vi "Periodic Tasks.vi"(8 "error in":errorcluster) -> ()   [LabVIEW 2017]
doc: "This VI runs in parallel to other tasks. It can contain as many user-defined periodic loops as you need. These can carry out PID or other sorts of timed response."
uses:
  Public/Documents/Cross The Road Electronics/Phoenix-LabVIEW/Motor Controller/Controls/CTRE_Phoenix_MotorControl_ControlMode.ctl
  Public/Documents/Cross The Road Electronics/Phoenix-LabVIEW/Motor Controller/Controls/CTRE_Phoenix_MotorControl_FeedbackDevice.ctl
  <vilib>/Rock Robotics/WPI/Utilities/WPI_GetSetVariantRefNum.vi
  Public/Documents/Cross The Road Electronics/Phoenix-LabVIEW/Motor Controller/Get/CTRE_Phoenix_MotorController_GetSelectedSensorData.vi
  Public/Documents/Cross The Road Electronics/Phoenix-LabVIEW/Motor Controller/Get/CTRE_Phoenix_MotorController_GetClosedLoopData.vi
panel:
  out "Error":T1(graph)
  in  "Left Phase":bool
  in  "Right Phase":bool
  in  "Setpoint":dbl
  in  "Control Mode":T2 items=["PercentOutput"=0, "Position"=1, "Velocity"=2, "Current"=3, "Follower"=5, "MotionProfile"=6, "MotionMagic"=7, "MotionMagicArc"=8, "MotionProfileArc"=10, "Disabled"=15]
  in  "Run PID":bool
  in  "Motion Magic":T3
  in  "Constants":cluster{"P":dbl, "I":dbl, "D":dbl, "F":dbl}
  in  "Change PID Constants":bool=TRUE
  in  "Zero Drive Sensors":bool
  out "Position":T4(graph)
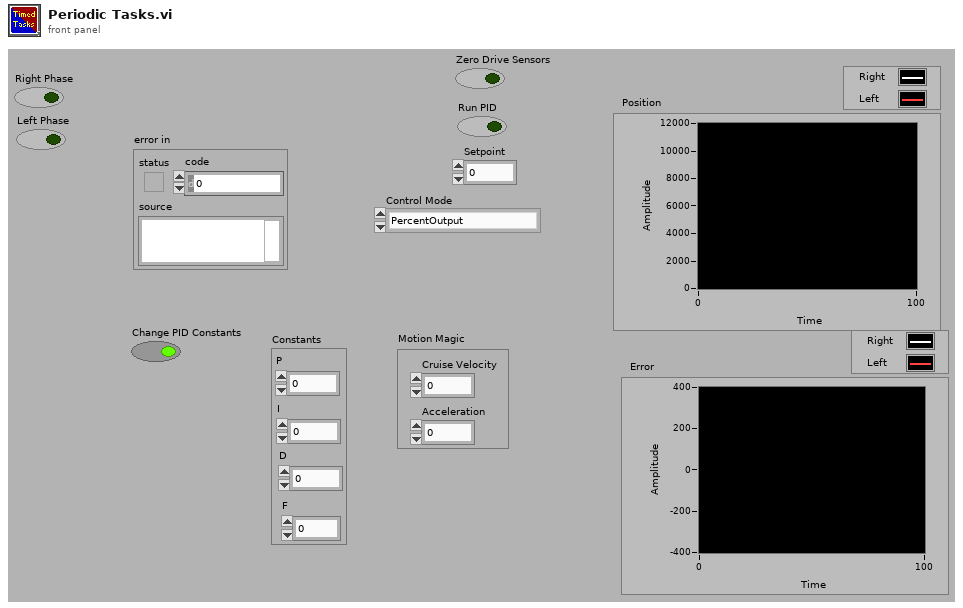
[diagram p1: front panel]
types:
  T1 = cluster{"Closed-loop Error":dbl, "Closed-loop Error":dbl}
  T2 = typedef "CTRE_Phoenix_MotorControl_ControlMode.ctl" = u16
  T3 = cluster{"Cruise Velocity":dbl, "Acceleration":dbl}
  T4 = cluster{"Position (Raw Sensor Units)":i32, "Position (Raw Sensor Units)":i32}
  T5 = typedef "CTRE_Phoenix_MotorControl_FeedbackDevice.ctl" = i8
  T6 = typedef "WPI_JoystickDevRef.ctl" = cluster{"Device":T7}
  T7 = typedef "WPI_JoystickDeviceEnum.ctl" = enum16{"USB 0", "USB 1", "USB 2", "USB 3", "USB 4", "USB 5"}
  T8 = typedef "WPI_MotorControlDeviceRef.ctl" = cluster{"DeviceStatus":errorcluster, "Type":T9, "PWM":cluster{"PWM Channel":T10, "DeadBand":T11}, "CAN":cluster{"Device Number":u8, "SetOutput VI Ref":variant, "GetOutput VI Ref":variant, "Enable VI Ref":variant, "Disable VI Ref":variant, "Data":variant}, "Invert":bool, "DIO PWM":cluster{"PWM \"Enable\" Channel":T10, "DIOChannel":T12, "PWM Rate":dbl}}
  T9 = typedef "WPI_MotorControlType.ctl" = enum16{"PWM", "CAN", "DIO PWM"}
  T10 = typedef "FPGA_DIOPWMChannel.ctl" = enum8{"PWM 0", "PWM 1", "PWM 2", "PWM 3", "PWM 4", "PWM 5", "PWM 6", "PWM 7", "PWM 8", "PWM 9", "PWM MXP 0", "PWM MXP 1", "PWM MXP 2", "PWM MXP 3", "PWM MXP 4", "PWM MXP 5", "PWM MXP 6", "PWM MXP 7", "PWM MXP 8", "PWM MXP 9", "Invalid"}
  T11 = typedef "WPI_PWMDeadband.ctl" = cluster{"Name":string, "maxPositivePwm":i32, "minPositivePwm":i32, "centerPwm":i32, "maxNegativePwm":i32, "minNegativePwm":i32, "angularRange":u16}
  T12 = typedef "FPGA_DIOChannel.ctl" = enum8{"DIO 0", "DIO 1", "DIO 2", "DIO 3", "DIO 4", "DIO 5", "DIO 6", "DIO 7", "DIO 8", "DIO 9", "DIO MXP 0", "DIO MXP 1", "DIO MXP 2", "DIO MXP 3", "DIO MXP 4", "DIO MXP 5", "DIO MXP 6", "DIO MXP 7", "DIO MXP 8", "DIO MXP 9", "DIO MXP 10", "DIO MXP 11", "DIO MXP 12", "DIO MXP 13", "DIO MXP 14", "DIO MXP 15", "SPI Port CS1", "SPI Port CS2", "SPI Port CS3", "SPI Port MISO", "SPI Port MOSI", "Invalid"}
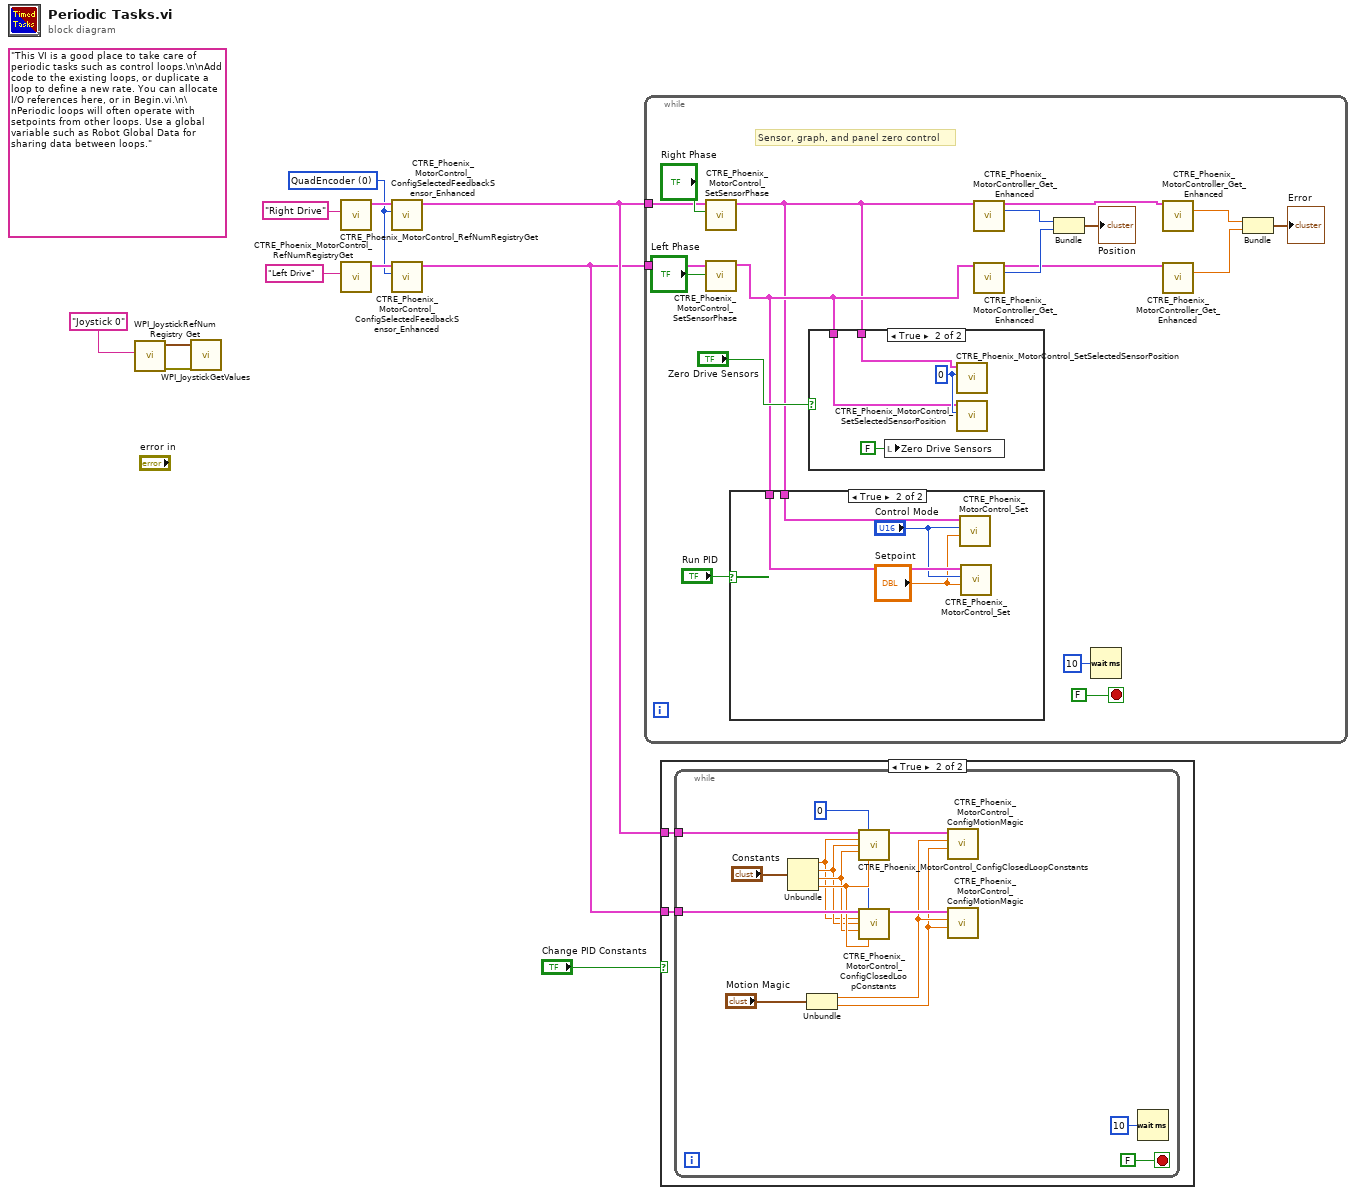
[diagram p0: block diagram]
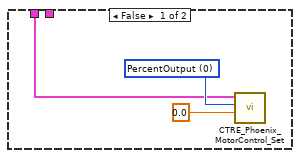
[diagram p3: hidden frame]
diagram:
  w4 = T5 0 items=["None"=-1, "QuadEncoder"=0, "Analog"=2, "Tachometer"=4, "Pulse Width Encoded Position"=8, "Sensor Sum (S0 + S1)"=9, "Sensor Difference (D0 - D1)"=10, "Remote Source 0"=11, "Remote Source 1"=12, "Software Emulated"=15] ("Feedback Device")
  (unwired) "This VI is a good place to take care of periodic tasks such as control loops.\n\nAdd code to the existing loops, or duplicate a loop to define a new rate. You can allocate I/O references here, or in Begin.vi.\n\nPeriodic loops will often operate with setpoints from other loops. Use a global variable such as Robot Global Data for sharing data between loops."
  n1 = call <vilib>:"WPI_JoystickRefNum Registry Get.vi"("refnum name"="Joystick 0") -> ("error out"=w10:errorcluster, "JoystickDevRef"=w9:T6)  [unwired: 1 in, 8 out]
  n2 = call <vilib>:"WPI_JoystickGetValues.vi"("error in (no error)"=w10, "JoystickDevRef"=w9) -> ()  [unwired: 5 in, 5 out]
  n3 = call "CTRE_Phoenix_MotorControl_RefNumRegistryGet.vi"("refnum name"="Right Drive") -> ("PhoenixMotorControlDevRef"=w7:T8)  [unwired: 9 in, 1 out]
  n4 = call "CTRE_Phoenix_MotorControl_RefNumRegistryGet.vi"("refnum name"="Left Drive") -> ("PhoenixMotorControlDevRef"=w8:T8)  [unwired: 9 in, 1 out]
  n5 = call "CTRE_Phoenix_MotorControl_ConfigSelectedFeedbackSensor_Enhanced.vi"("Feedback Device"=w4, "PhoenixMotorControlDevRef"=w7) -> ("PhoenixMotorControlDevRef"=w2:T8)  [unwired: 8 in, 1 out]
  n6 = call "CTRE_Phoenix_MotorControl_ConfigSelectedFeedbackSensor_Enhanced.vi"("Feedback Device"=w4, "PhoenixMotorControlDevRef"=w8) -> ("PhoenixMotorControlDevRef"=w1:T8)  [unwired: 8 in, 1 out]
  n7 = while {
    tunnel: w1 -> [w21]
    tunnel: w2 -> [w19]
    stop <- FALSE stop-if-true
    # "Sensor, graph, and panel zero control"
    n8 = call "CTRE_Phoenix_MotorControl_SetSensorPhase.vi"("PhaseSensor"="Right Phase", "PhoenixMotorControlDevRef"=w19) -> ("PhoenixMotorControlDevRef"=w12:T8)  [unwired: 8 in, 1 out]
    n9 = call "CTRE_Phoenix_MotorControl_SetSensorPhase.vi"("PhaseSensor"="Left Phase", "PhoenixMotorControlDevRef"=w21) -> ("PhoenixMotorControlDevRef"=w18:T8)  [unwired: 8 in, 1 out]
    n10 = case shown="True" "Run PID" {
      tunnel: w18 -> [w30 w36]
      tunnel: w12 -> [_ w33]
      frame False {
        w32 = T2 0 items=["PercentOutput"=0, "Position"=1, "Velocity"=2, "Current"=3, "Follower"=5, "MotionProfile"=6, "MotionMagic"=7, "MotionMagicArc"=8, "MotionProfileArc"=10, "Disabled"=15] ("Control Mode 2")
        n11 = call "CTRE_Phoenix_MotorControl_Set.vi"("Output"=0.0 ("Output 2"), "Control Mode"=w32, "PhoenixMotorControlDevRef"=w30) -> ()  [unwired: 7 in, 2 out]
      }
      frame True {
        n12 = call "CTRE_Phoenix_MotorControl_Set.vi"("Output"="Setpoint", "Control Mode"="Control Mode", "PhoenixMotorControlDevRef"=w33) -> ()  [unwired: 7 in, 2 out]
        n13 = call "CTRE_Phoenix_MotorControl_Set.vi"("Output"="Setpoint", "Control Mode"="Control Mode", "PhoenixMotorControlDevRef"=w36) -> ()  [unwired: 7 in, 2 out]
      }
    }
    n14 = case shown="True" "Zero Drive Sensors" {
      tunnel: w12 -> [_ w39]
      tunnel: w18 -> [_ w38]
      frame False {
      }
      frame True {
        w40 = 0 ("New Sensor Position")
        n15 = local write "Zero Drive Sensors"(FALSE ("Zero Drive Sensors")) -> ()
        n16 = call "CTRE_Phoenix_MotorControl_SetSelectedSensorPosition.vi"("New Sensor Position"=w40, "PhoenixMotorControlDevRef"=w39) -> ()  [unwired: 8 in, 2 out]
        n17 = call "CTRE_Phoenix_MotorControl_SetSelectedSensorPosition.vi"("New Sensor Position"=w40, "PhoenixMotorControlDevRef"=w38) -> ()  [unwired: 8 in, 2 out]
      }
    }
    n18 = call-poly "CTRE_Phoenix_MotorController_Get_Enhanced.vi"("PhoenixMotorControlDevRef"=w12) -> ("PhoenixMotorControlDevRef"=w14:T8, "Position (Raw Sensor Units)"=w27:i32)  [unwired: 11 in, 2 out]
    n19 = call-poly "CTRE_Phoenix_MotorController_Get_Enhanced.vi"("PhoenixMotorControlDevRef"=w18) -> ("PhoenixMotorControlDevRef"=w13:T8, "Position (Raw Sensor Units)"=w26:i32)  [unwired: 11 in, 2 out]
    n20 = Bundle("Position (Raw Sensor Units)"=w27, "Position (Raw Sensor Units)"=w26) -> (→"Position":T4)  [unwired: 1 in]
    n21 = Wait (ms)(milliseconds to wait=u32 10) -> ()  [unwired: 1 out]
    n22 = call-poly "CTRE_Phoenix_MotorController_Get_Enhanced.vi"("PhoenixMotorControlDevRef"=w14) -> ("Closed-loop Error"=w15:dbl)  [unwired: 10 in, 4 out]
    n23 = call-poly "CTRE_Phoenix_MotorController_Get_Enhanced.vi"("PhoenixMotorControlDevRef"=w13) -> ("Closed-loop Error"=w16:dbl)  [unwired: 10 in, 4 out]
    n24 = Bundle("Closed-loop Error"=w15, "Closed-loop Error"=w16) -> (→"Error":T1)  [unwired: 1 in]
  }
  n25 = case shown="True" "Change PID Constants" {
    tunnel: w2 -> [_ w42]
    tunnel: w1 -> [_ w41]
    frame False {
    }
    frame True {
      n26 = while {
        tunnel: w42 -> [w55]
        tunnel: w41 -> [w53]
        stop <- FALSE stop-if-true
        w43 = 0 ("slotIdx")
        n27 = Unbundle("Constants") -> ("P"=w49:dbl, "I"=w50:dbl, "D"=w51:dbl, "F"=w52:dbl)
        n28 = Unbundle("Motion Magic") -> ("Cruise Velocity"=w45:dbl, "Acceleration"=w44:dbl)
        n29 = call "CTRE_Phoenix_MotorControl_ConfigClosedLoopConstants.vi"("PhoenixMotorControlDevRef"=w55, "slotIdx"=w43, "P"=w49, "I"=w50, "D"=w51, "F"=w52) -> ("PhoenixMotorControlDevRef"=w48:T8)  [unwired: 8 in, 1 out]
        n30 = call "CTRE_Phoenix_MotorControl_ConfigClosedLoopConstants.vi"("PhoenixMotorControlDevRef"=w53, "slotIdx"=w43, "P"=w49, "I"=w50, "D"=w51, "F"=w52) -> ("PhoenixMotorControlDevRef"=w47:T8)  [unwired: 8 in, 1 out]
        n31 = call "CTRE_Phoenix_MotorControl_ConfigMotionMagic.vi"("Acceleration"=w44, "Cruise Velocity"=w45, "PhoenixMotorControlDevRef"=w48) -> ()  [unwired: 7 in, 2 out]
        n32 = call "CTRE_Phoenix_MotorControl_ConfigMotionMagic.vi"("Acceleration"=w44, "Cruise Velocity"=w45, "PhoenixMotorControlDevRef"=w47) -> ()  [unwired: 7 in, 2 out]
        n33 = Wait (ms)(milliseconds to wait=u32 10) -> ()  [unwired: 1 out]
      }
    }
  }
